vi "Configure ARB Function Shape.vi"(8 "error in (no error)":errorcluster, 10 "Type(0:Pulse)":u16(ring) items=["PULSe", "SINusiod", "UDEFined", "CDWell", "SEQuence"], 11 "VISA resource name":refnum<visa-resource-name>) -> (0 "error out":errorcluster, 3 "VISA resource name out":refnum<visa-resource-name>)   [LabVIEW 2015, in "IT6000C.lvlib"]
doc: "This command sets the functionality of the ARB.\n\n<b>Type</b>\n0:PULSe\n1:SINusiod\n2:UDEFined\n3:CDWell\n4:SEQuence"
uses:
  <instrlib>/IT6000C/IT6000C.lvlib
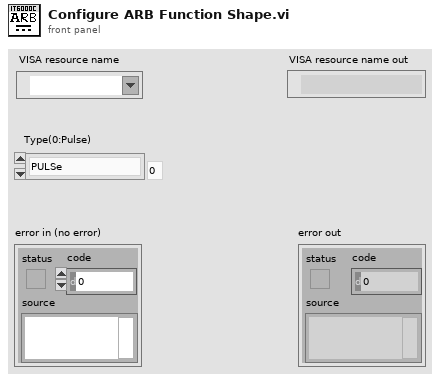
[diagram p1: front panel]
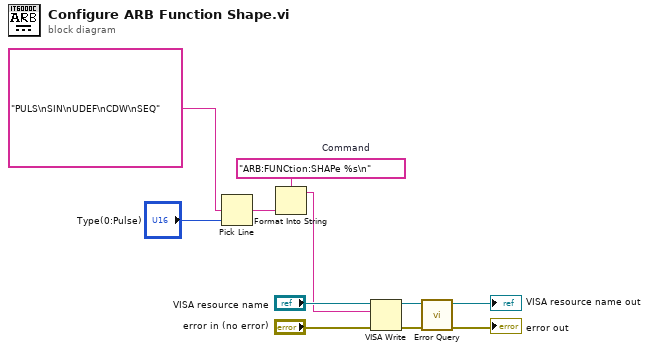
[diagram p0: block diagram]
diagram:
  w5 = "ARB:FUNCtion:SHAPe %s\n"  # Command
  n1 = Pick Line(multi-line string="PULS\nSIN\nUDEF\nCDW\nSEQ", line index="Type(0:Pulse)") -> (output string=w1:string)  [unwired: 1 in]
  n2 = Format Into String(format string=w5, w1) -> (resulting string=w4:string)  [unwired: 2 in, 1 out]
  n3 = VISA Write(VISA resource name="VISA resource name", write buffer=w4, error in (no error)="error in (no error)") -> (VISA resource name out=w8:refnum<visa-resource-name>, error out=w9:errorcluster)  [unwired: 1 out]
  n4 = call <instrlib>:"Error Query.vi"("error in (no error)"=w9, "VISA resource name"=w8) -> ("error out"=→"error out":errorcluster, "VISA resource name out"=→"VISA resource name out":refnum<visa-resource-name>)  [unwired: 6 in, 2 out]
